vi "dbsys_test.vi"(0 "nominal":dbl, 1 "delta":dbl, 2 "actualValue":dbl, 3 "boundaryValue":dbl, 4 "tsIndex":string, 5 "status":bool, 7 "decimalsAreNulls":bool) -> (6 "Статус":i32)   [LabVIEW 2017]
uses:
  DBSysCore.dll
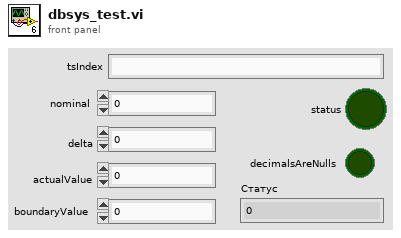
[diagram p1: front panel]
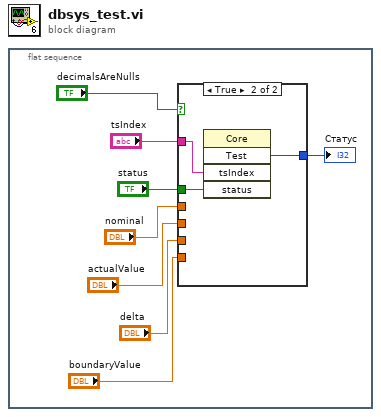
[diagram p0: block diagram]
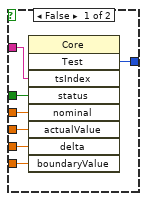
[diagram p2: hidden frame]
diagram:
  n1 = flat-sequence {
    frame #0 {
      n2 = case shown="True" "decimalsAreNulls" {
        tunnel: "tsIndex" -> [w14 w18]
        tunnel: "status" -> [w15 w17]
        tunnel: "nominal" -> [w13 _]
        tunnel: "actualValue" -> [w12 _]
        tunnel: "delta" -> [w11 _]
        tunnel: "boundaryValue" -> [w10 _]
        tunnel: [w9 w16] -> w8
        frame False {
          n3 = invoke class="Core" method="Test"("tsIndex"=w14, "status"=w15, "nominal"=w13, "actualValue"=w12, "delta"=w11, "boundaryValue"=w10) -> ("Test"=w9:i32)  [unwired: 3 in, 8 out]
        }
        frame True {
          n4 = invoke class="Core" method="Test"("tsIndex"=w18, "status"=w17) -> ("Test"=w16:i32)  [unwired: 3 in, 4 out]
        }
      }
      "Статус" <- w8
    }
  }
